vi "Teleop.vi"(10 "Match Info":T1={"Autonomous Elapsed Seconds"=0.0, "TeleOp Elapsed Seconds"=0.0, "Disabled Elapsed Seconds"=0.0, "Visited Autonomous"=FALSE, "Visited TeleOp"=FALSE, "Visited Disabled"=FALSE, "Autonomous Settings"={"Autonomous Style"=enum."Independent", "VI Refnum"=refnum}}, 11 "Call Context":T2) -> ()   [LabVIEW 2012]
doc: "This VI is called for each TeleOp packet received from the DS where the robot is not disabled. It is often used to read from the joysticks and update I/O or to update setpoints for timed control loops. It should complete and return within 20 milliseconds or it may miss DS packets."
uses:
  <vilib>/Rock Robotics/WPI/DriverStation/WPI_DriverStationDerivedRobotMode.ctl
  <vilib>/Rock Robotics/WPI/DriverStation/WPI_DriverStationMatch Info.ctl
  Robot Global Data.vi
  SubVI/Global 1 (shooter controls).vi
  SubVI/grabber control buttons.vi
  <vilib>/Rock Robotics/WPI/RobotDrive/WPI_RobotDriveMecanumDrive_Cartesian.vi
  <vilib>/Rock Robotics/WPI/Joystick/WPI_JoystickGetSetRefNum.vi
  <vilib>/Rock Robotics/WPI/RobotDrive/WPI_RobotDriveGetSetRefNum.vi
panel:
  out "br":dbl
  out "bl":dbl
  out "fr":dbl
  out "fl":dbl
  out "potvalue":dbl
  out "Axis 3 (throttle) 2":dbl
  out "Axis 3 (throttle)":dbl
  out "Numeric 1":dbl(slide) scale=0.0..100.0
  out "Boolean 2":bool
  out "Boolean 1":bool
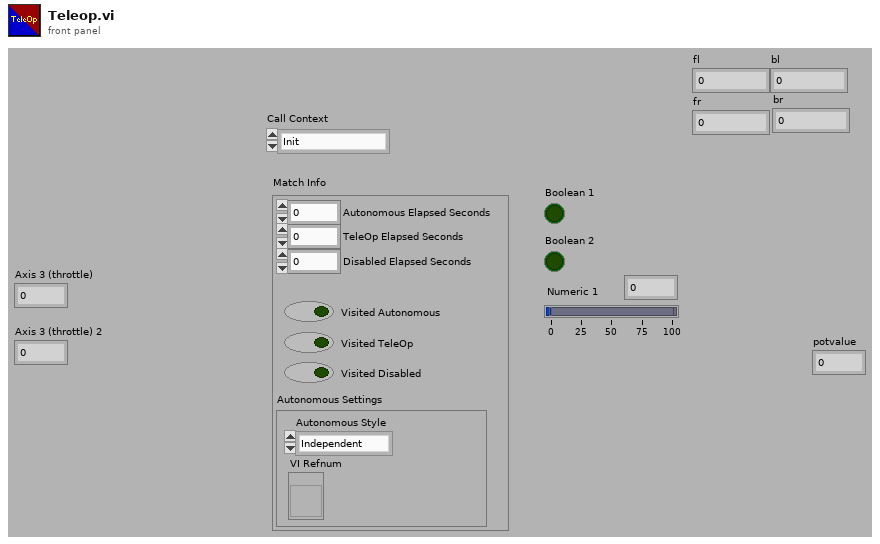
[diagram p1: front panel]
types:
  T1 = typedef "WPI_DriverStationMatch Info.ctl" = cluster{"Autonomous Elapsed Seconds":dbl, "TeleOp Elapsed Seconds":dbl, "Disabled Elapsed Seconds":dbl, "Visited Autonomous":bool, "Visited TeleOp":bool, "Visited Disabled":bool, "Autonomous Settings":cluster{"Autonomous Style":enum16{"Iterative", "Independent"}, "VI Refnum":refnum<vi>}}
  T2 = typedef "WPI_DriverStationDerivedRobotMode.ctl" = enum16{"Init", "Execute", "Stop"}
  T3 = typedef "WPI_JoystickDevRef.ctl" = cluster{"Device":T4}
  T4 = typedef "WPI_JoystickDeviceEnum.ctl" = enum16{"USB 1", "USB 2", "USB 3", "USB 4", "Kinect 1", "Kinect 2"}
  T5 = typedef "WPI_JoystickButtonState.ctl" = cluster{"Button 1":bool, "Button 2":bool, "Button 3":bool, "Button 4":bool, "Button 5":bool, "Button 6":bool, "Button 7":bool, "Button 8":bool, "Button 9":bool, "Button 10":bool, "Button 11":bool, "Button 12":bool}
  T6 = cluster{"axis 1 (x)":dbl, "axis 2 (y)":dbl, "axis 3 (throttle)":dbl, "axis 4":dbl, "axis 5":dbl, "axis 6":dbl}
  T7 = cluster{"pickupoveride":bool, "stophunting?":bool, "wanthunt?":bool}
  T8 = typedef "WPI_RobotDriveDevRef.ctl" = cluster{"DevStatus":errorcluster, "Motors[]":T9[], "Square Inputs":bool, "Max Output":dbl, "Isochronous":bool}
  T9 = typedef "WPI_MotorControlDeviceRef.ctl" = cluster{"DeviceStatus":errorcluster, "Type":enum16{"PWM", "CAN"}, "PWM":cluster{"Digital Module":T10, "PWM Channel":T11, "DeadBand":T12}, "CAN":cluster{"Device Number":u8, "Control Mode":T13, "Semaphore":T14, "Max Vout":dbl}, "Invert":bool, "TransformRef":T15, "InvTransformRef":T15}
  T10 = typedef "FPGA_TypedefDigitalModule.ctl" = enum16{"Digital Module 1", "Digital Module 2"}
  T11 = typedef "FPGA_DIOPWMChannel.ctl" = enum8{"PWM 1", "PWM 2", "PWM 3", "PWM 4", "PWM 5", "PWM 6", "PWM 7", "PWM 8", "PWM 9", "PWM 10", "Invalid"}
  T12 = typedef "WPI_PWMDeadband.ctl" = cluster{"Name":string, "maxPositivePwm":i32, "minPositivePwm":i32, "centerPwm":i32, "maxNegativePwm":i32, "minNegativePwm":i32, "angularRange":u16}
  T13 = typedef "WPI_CANJaguar_ControlMode.ctl" = enum8{"Percent VBus", "Current", "Speed", "Position", "Voltage"}
  T14 = typedef "Semaphore RefNum" = refnum<k1>
  T15 = typedef "WPI_PWMTransform_ConPane.ctl" = refnum<vi>
  T16 = typedef "WPI_EncoderDevRef.ctl" = cluster{"DevStatus":errorcluster, "EncoderIndex":T17, "CounterIndex":T18, "DistancePerCount":dbl, "Decoding Type":T19}
  T17 = typedef "FPGA_EncoderIdx.ctl" = enum8{"Enc 0", "Enc 1", "Enc 2", "Enc 3", "Invalid"}
  T18 = typedef "FPGA_CounterCtrSystemIndex.ctl" = enum8{"Ctr 0", "Ctr 1", "Ctr 2", "Ctr 3", "Ctr 4", "Ctr 5", "Ctr 6", "Ctr 7", "Invalid"}
  T19 = typedef "WPI_EncoderType.ctl" = enum16{"1x", "2x", "4x"}
  T20 = typedef "WPI_AnalogChannelDevRef.ctl" = cluster{"DevStatus":errorcluster, "Analog Module":T21, "Analog Channel":T22}
  T21 = typedef "FPGA_TypedefAnalogModule.ctl" = enum16{"Analog Module 1", "Analog Module 2"}
  T22 = typedef "FPGA_AIChannel.ctl" = enum8{"AI 1", "AI 2", "AI 3", "AI 4", "AI 5", "AI 6", "AI 7", "AI 8", "Invalid"}
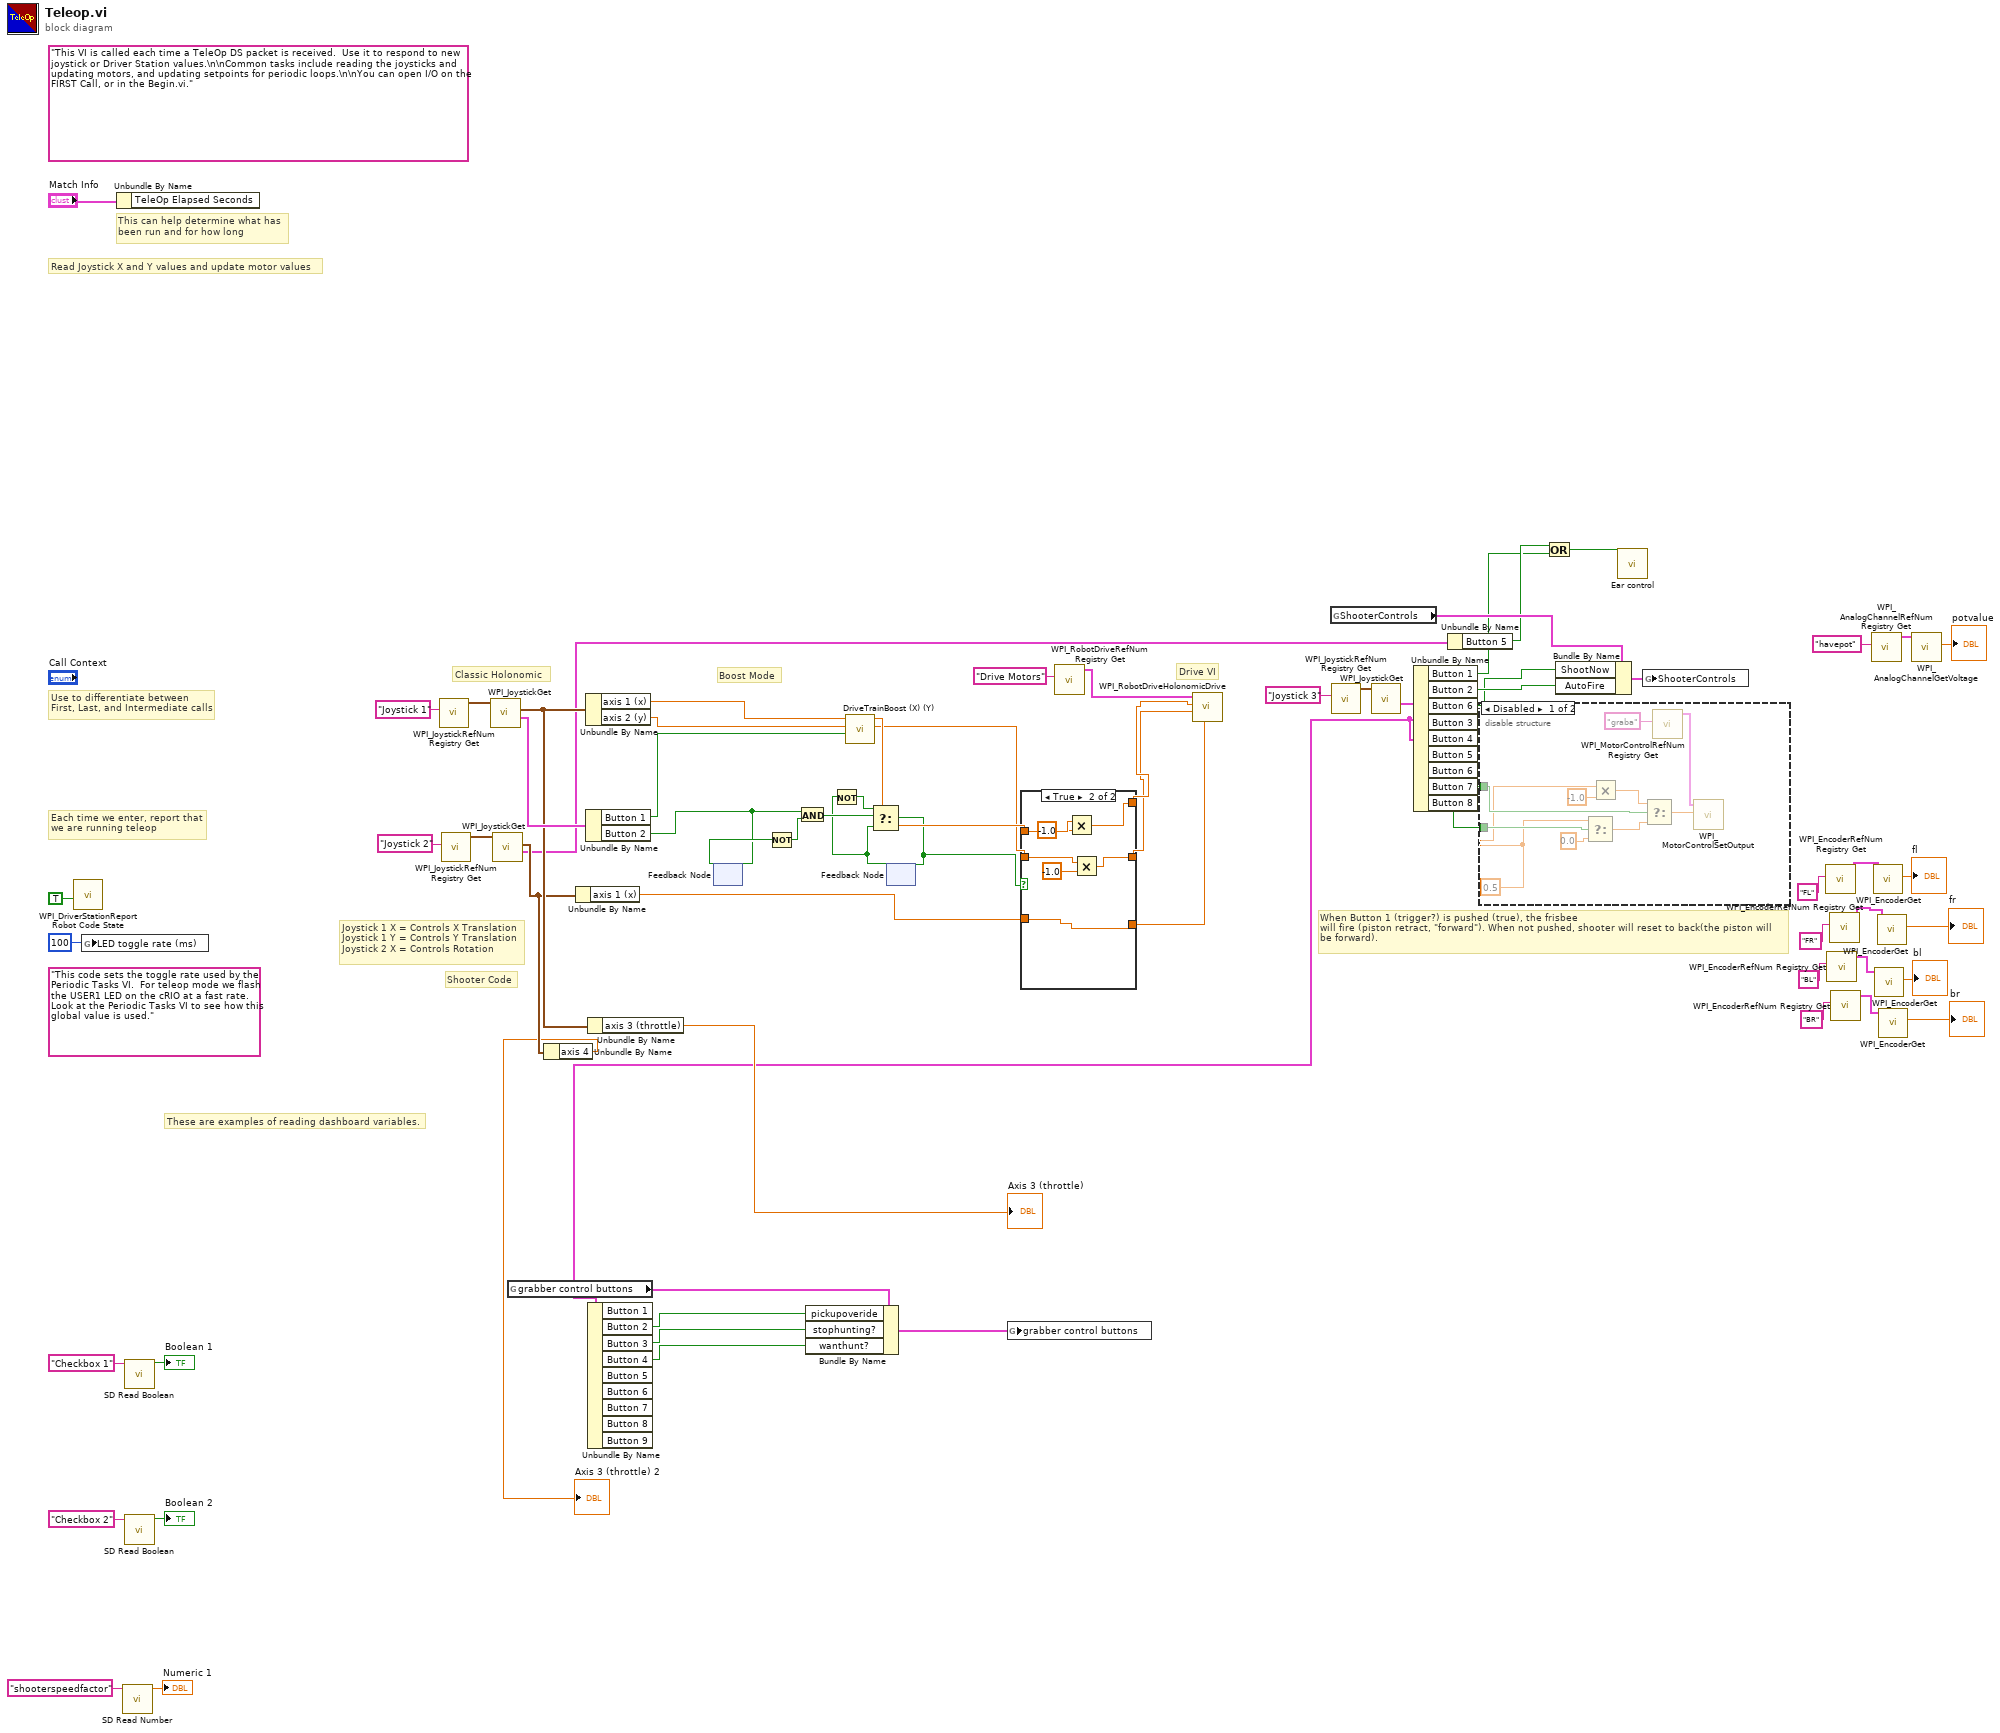
[diagram p0: block diagram]
diagram:
  (unwired) "This code sets the toggle rate used by the Periodic Tasks VI.  For teleop mode we flash the USER1 LED on the cRIO at a fast rate.  Look at the Periodic Tasks VI to see how this global value is used."
  (unwired) "This VI is called each time a TeleOp DS packet is received.  Use it to respond to new joystick or Driver Station values.\n\nCommon tasks include reading the joysticks and updating motors, and updating setpoints for periodic loops.\n\nYou can open I/O on the FIRST Call, or in the Begin.vi."
  # "When Button 1 (trigger?) is pushed (true), the frisbee\nwill fire (piston retract, \"forward\"). When not pushed, shooter will reset to back(the piston will\nbe forward)."
  # "Shooter Code"
  # "Drive VI"
  # "Joystick 1 X = Controls X Translation\nJoystick 1 Y = Controls Y Translation\nJoystick 2 X = Controls Rotation"
  # "Boost Mode"
  # "Classic Holonomic"
  # "These are examples of reading dashboard variables."
  # "Each time we enter, report that\nwe are running teleop"
  # "Use to differentiate between\nFirst, Last, and Intermediate calls"
  # "This can help determine what has\nbeen run and for how long"
  # "Read Joystick X and Y values and update motor values"
  n1 = call <vilib>:"WPI_DriverStationReport Robot Code State.vi"("TeleOp"=TRUE ("Autonomous")) -> ()  [unwired: 10 in, 1 out]
  n2 = global write "Robot Global Data.vi" "LED toggle rate (ms)"(u32 100 ("LED ms toggle rate")) -> ()
  n3 = Unbundle By Name("Match Info") -> ()  [unwired: 1 out]
  n4 = call <vilib>:"SD Read Number.vi"("Name"="shooterspeedfactor" ("refnum name")) -> ("Numeric"=→"Numeric 1":dbl)  [unwired: 8 in, 2 out]
  n5 = call <vilib>:"SD Read Boolean.vi"("Name"="Checkbox 1" ("refnum name")) -> ("Boolean"=→"Boolean 1":bool)  [unwired: 8 in, 2 out]
  n6 = call <vilib>:"SD Read Boolean.vi"("Name"="Checkbox 2" ("refnum name")) -> ("Boolean"=→"Boolean 2":bool)  [unwired: 8 in, 2 out]
  n7 = call <vilib>:"WPI_JoystickRefNum Registry Get.vi"("refnum name"="Joystick 1") -> ("JoystickDevRef"=w61:T3)  [unwired: 1 in, 9 out]
  n8 = call <vilib>:"WPI_JoystickRefNum Registry Get.vi"("refnum name"="Joystick 2") -> ("JoystickDevRef"=w60:T3)  [unwired: 1 in, 9 out]
  n9 = call <vilib>:"WPI_JoystickGet.vi"("JoystickDevRef"=w61) -> ("Buttons"=w55:T5, "Axes"=w51:T6)  [unwired: 1 in, 4 out]
  n10 = call <vilib>:"WPI_JoystickGet.vi"("JoystickDevRef"=w60) -> ("Buttons"=w8:T5, "Axes"=w49:T6)  [unwired: 1 in, 4 out]
  n11 = global read "grabber control buttons.vi" "grabber control buttons"() -> (w29:T7)
  n12 = Unbundle By Name(w49) -> ("axis 4"=→"Axis 3 (throttle) 2":dbl)
  n13 = Unbundle By Name(w49) -> ("axis 1 (x)"=w44:dbl)
  n14 = Unbundle By Name(w51) -> ("axis 1 (x)"=w53:dbl, "axis 2 (y)"=w52:dbl)
  n15 = Unbundle By Name(w55) -> ("Button 1"=w54:bool, "Button 2"=w1:bool)
  n16 = Unbundle By Name(w51) -> ("axis 3 (throttle)"=→"Axis 3 (throttle)":dbl)
  n17 = feedback #1() -> (w6:bool)  [unwired: 1 in]
  n18 = feedback-in #1(w1) -> ()
  n19 = Not(x=w6) -> (.not. x?=w7:bool)
  n20 = And(x=w1, y=w7) -> (x .and. y?=w5:bool)
  n21 = call "DriveTrainBoost (X) (Y).vi"("Boost on"=w54, "axis 2 (y) in"=w52, "axis 1 (x) in"=w53) -> ("axis 2 (y) out"=w45:dbl, "axis 1 (x) out"=w48:dbl)  [unwired: 7 in]
  n22 = feedback #2() -> (w3:bool)  [unwired: 1 in]
  n23 = Not(x=w3) -> (.not. x?=w4:bool)
  n24 = Select(t=w4, s=w5, f=w3) -> (s? t:f=w2:bool)
  n25 = feedback-in #2(w2) -> ()
  n26 = case shown="True" w2 {
    tunnel: w48 -> [w72 w78]
    tunnel: [w72 w75] -> w47
    tunnel: [w71 w74] -> w46
    tunnel: w45 -> [w71 w79]
    tunnel: w44 -> [w70 w73]
    tunnel: [w70 w73] -> w43
    frame False {
    }
    frame True {
      n27 = Multiply(x=w78, y=-1.0) -> (x*y=w75:dbl)
      n28 = Multiply(x=w79, y=-1.0) -> (x*y=w74:dbl)
    }
  }
  n29 = call <vilib>:"WPI_RobotDriveRefNum Registry Get.vi"("refnum name"="Drive Motors") -> ("RobotDriveDevRef"=w57:T8)  [unwired: 9 in, 1 out]
  n30 = call-poly <vilib>:"WPI_RobotDriveHolonomicDrive.vi"("Rotation"=w43, "Y"=w46, "X"=w47, "RobotDriveDevRef"=w57) -> ()  [unwired: 5 in, 3 out]
  n31 = global read "Global 1 (shooter controls).vi" "ShooterControls"() -> (w37:cluster{"ShootNow":bool, "AutoFire":bool})
  n32 = call <vilib>:"WPI_JoystickRefNum Registry Get.vi"("refnum name"="Joystick 3") -> ("JoystickDevRef"=w39:T3)  [unwired: 9 in, 1 out]
  n33 = call <vilib>:"WPI_JoystickGet.vi"("JoystickDevRef"=w39) -> ("Buttons"=w12:T5)  [unwired: 4 in, 2 out]
  n34 = Unbundle By Name(w12) -> ("Button 2"=w11:bool, "Button 3"=w10:bool, "Button 4"=w9:bool)  [unwired: 6 out]
  n35 = Bundle By Name(cluster=w29, "pickupoveride"=w11, "stophunting?"=w10, "wanthunt?"=w9) -> (w30:T7)
  n36 = global write "grabber control buttons.vi" "grabber control buttons"(w30) -> ()
  n37 = Unbundle By Name(w12) -> ("Button 1"=w25:bool, "Button 2"=w38:bool, "Button 6"=w28:bool, "Button 7"=w27:bool, "Button 8"=w26:bool)  [unwired: 4 out]
  n38 = Unbundle By Name(w8) -> ("Button 5"=w35:bool)
  n39 = disable-structure shown="Disabled" {
    disable-tunnel: w27 -> [w82 _]
    disable-tunnel: w26 -> [w81 _]
    frame Disabled {
      w80 = 0.5 ("t")
      n40 = Select(t=w80, s=w81, f=0.0 ("Output")) -> (s? t:f=w83:dbl)
      n41 = Multiply(x=w80, y=-1.0 ("Output")) -> (x*y=w84:dbl)
      n42 = Select(t=w84, s=w82, f=w83) -> (s? t:f=w86:dbl)
      n43 = call <vilib>:"WPI_MotorControlRefNum Registry Get.vi"("refnum name"="graba") -> ("MotorControlDevRef"=w89:T9)  [unwired: 9 in, 1 out]
      n44 = call <vilib>:"WPI_MotorControlSetOutput.vi"("Output"=w86, "MotorControlDevRef"=w89) -> ()  [unwired: 7 in, 3 out]
    }
    frame Enabled {
    }
  }
  n45 = Or(x=w35, y=w25) -> (x .or. y?=w34:bool)
  n46 = Bundle By Name(cluster=w37, "ShootNow"=w28, "AutoFire"=w38) -> (w36:cluster{"ShootNow":bool, "AutoFire":bool})
  n47 = call "Ear control.vi"("Toggle Ears"=w34) -> ()  [unwired: 11 in]
  n48 = global write "Global 1 (shooter controls).vi" "ShooterControls"(w36) -> ()
  n49 = call <vilib>:"WPI_EncoderRefNum Registry Get.vi"("refnum name"="FL") -> ("EncoderDevRef"=w20:T16)  [unwired: 9 in, 1 out]
  n50 = call <vilib>:"WPI_EncoderRefNum Registry Get.vi"("refnum name"="BL") -> ("EncoderDevRef"=w21:T16)  [unwired: 9 in, 1 out]
  n51 = call <vilib>:"WPI_EncoderRefNum Registry Get.vi"("refnum name"="FR") -> ("EncoderDevRef"=w17:T16)  [unwired: 9 in, 1 out]
  n52 = call <vilib>:"WPI_EncoderRefNum Registry Get.vi"("refnum name"="BR") -> ("EncoderDevRef"=w24:T16)  [unwired: 9 in, 1 out]
  n53 = call <vilib>:"WPI_AnalogChannelRefNum Registry Get.vi"("refnum name"="havepot") -> ("AIDeviceRef"=w33:T20)  [unwired: 9 in, 1 out]
  n54 = call <vilib>:"WPI_EncoderGet.vi"("EncoderDevRef"=w20) -> ("Distance"=→"fl":dbl)  [unwired: 5 in, 5 out]
  n55 = call <vilib>:"WPI_EncoderGet.vi"("EncoderDevRef"=w21) -> ("Distance"=→"bl":dbl)  [unwired: 5 in, 5 out]
  n56 = call <vilib>:"WPI_EncoderGet.vi"("EncoderDevRef"=w17) -> ("Distance"=→"fr":dbl)  [unwired: 5 in, 5 out]
  n57 = call <vilib>:"WPI_EncoderGet.vi"("EncoderDevRef"=w24) -> ("Distance"=→"br":dbl)  [unwired: 5 in, 5 out]
  n58 = call <vilib>:"WPI_AnalogChannelGetVoltage.vi"("AIDeviceRef"=w33) -> ("Voltage"=→"potvalue":dbl)  [unwired: 8 in, 2 out]
